vi "Voltage Ramp Text Out.vi"(1 "VoltageRamp":T2={"VISA Resource Name"="", "extra wait"=1, "start"=1e-12, "end"=0.002, "Sweep Time (H:M:S)"=1800.0, "Log Linear"=FALSE, "interval(sec)"=0.5, "Select instrument"=enum."Yokogawa GS200 Coarse"} {"interval(sec)" min=0.5 step=0.1; "Sweep Time (H:M:S)" format="%<%H:%M:%S>t"; "extra wait" min=0; "start" format="%#.7e"; "end" format="%#.7e"}) -> (0 "Command text":string[][](array[string]))   [LabVIEW 2021]
uses:
  VoltageRamp.ctl
  VoltageRamp Instrument.ctl
panel:
  out "Select instrument 2":T1
  out "Sweep Time (H:M:S)":dbl
  out "String Cluster":T3
  # "Voltage Ramp"
  # "Select\nInstrument"
  # "Instrument \nAddress"
  # "Log"
  # "End Voltage (V)"
  # "Sweep Time (HH:MM:SS)"
  # "Start Voltage (V)"
  # "Linear"
  # "seconds"
  # "Minimum Time Interval Between Two Points"
  # "seconds"
  # "AND wait extra"
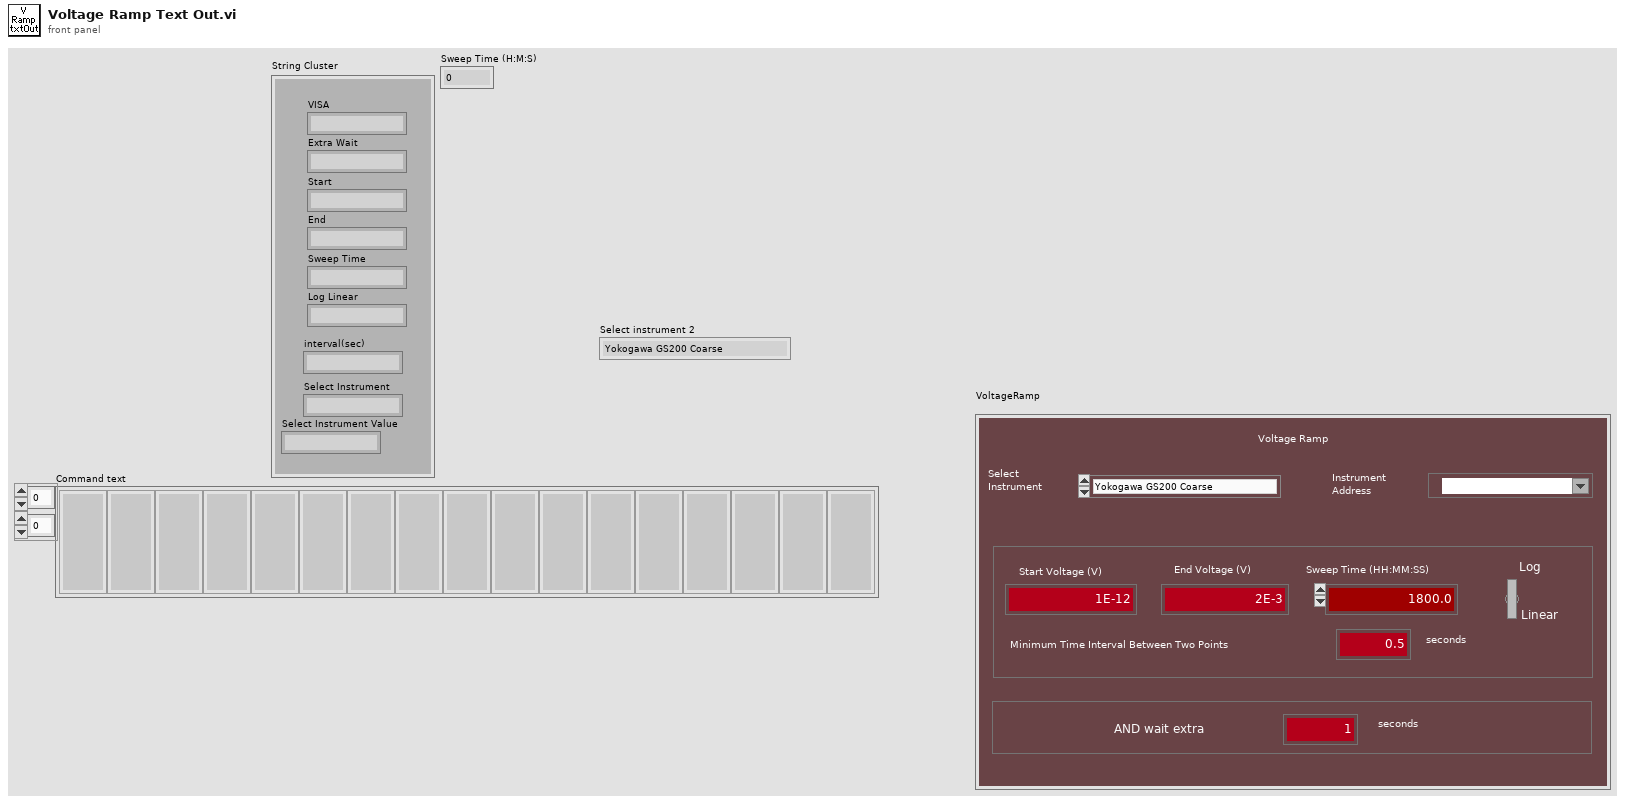
[diagram p1: front panel]
types:
  T1 = typedef "VoltageRamp Instrument.ctl" = enum16{"Yokogawa GS200 Coarse", "Keithley 24xx Coarse", "Keithley 230"}
  T2 = typedef "VoltageRamp.ctl" = cluster{"VISA Resource Name":refnum<visa-resource-name>, "extra wait":i32, "start":dbl, "end":dbl, "Sweep Time (H:M:S)":dbl, "Log Linear":bool, "interval(sec)":dbl, "Select instrument":T1}
  T3 = cluster{"VISA":string, "Extra Wait":string, "Start":string, "End":string, "Sweep Time":string, "Log Linear":string, "interval(sec)":string, "Select Instrument":string, "Select Instrument Value":string}
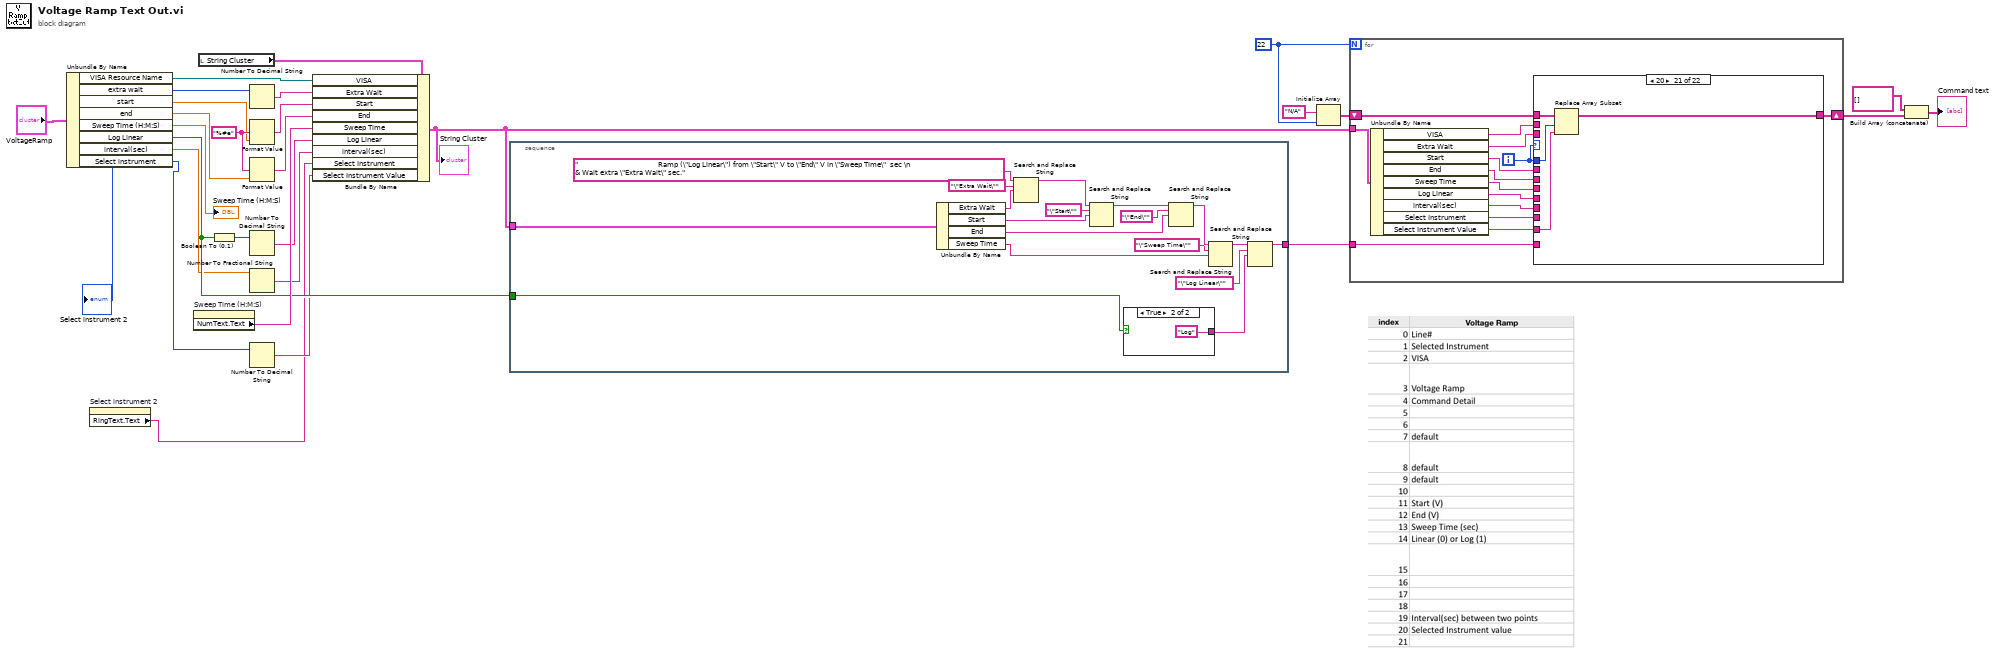
[diagram p0: block diagram]
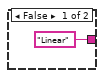
[diagram p2: hidden frame]
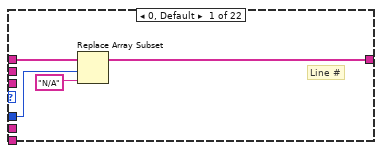
[diagram p3: hidden frame]
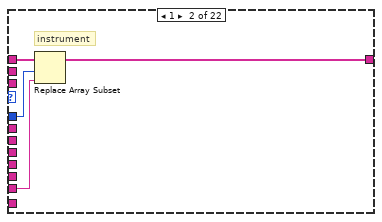
[diagram p4: hidden frame]
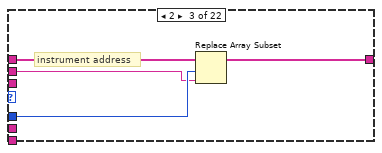
[diagram p5: hidden frame]
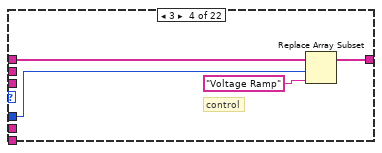
[diagram p6: hidden frame]
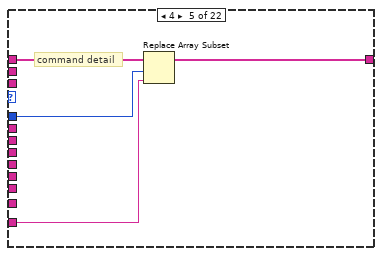
[diagram p7: hidden frame]
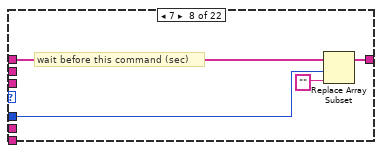
[diagram p10: hidden frame]
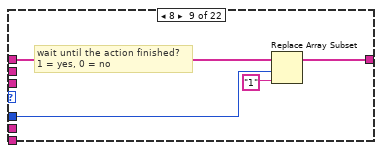
[diagram p11: hidden frame]
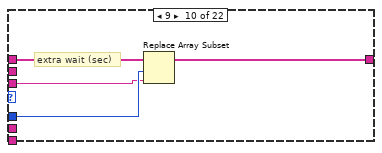
[diagram p12: hidden frame]
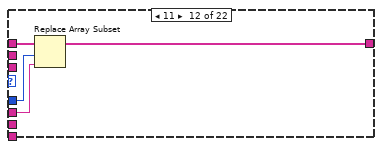
[diagram p14: hidden frame]
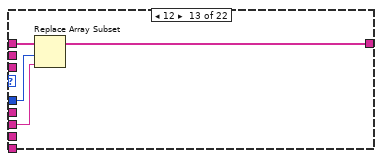
[diagram p15: hidden frame]
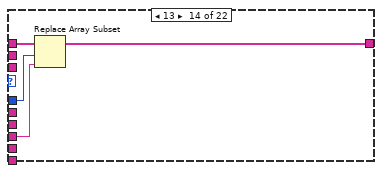
[diagram p16: hidden frame]
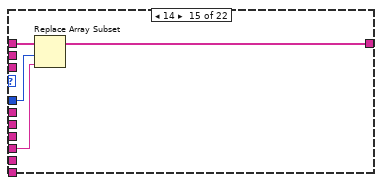
[diagram p17: hidden frame]
diagram:
  w17 = "%#e" ("format string")
  w25 = 22
  n1 = Unbundle By Name("VoltageRamp") -> ("VISA Resource Name"=w10:refnum<visa-resource-name>, "extra wait"=w12:i32, "start"=w15:dbl, "end"=w16:dbl, "Sweep Time (H:M:S)"=→"Sweep Time (H:M:S)":dbl, "Log Linear"=w8:bool, "interval(sec)"=w6:dbl, "Select instrument"=w1:T1)
  "Select instrument 2" <- w1
  n2 = property on="Select instrument 2" class="Enum (strict)"() -> ("RingText.Text"=w2:string)  [unwired: 2 in, 2 out]
  n3 = property on="Sweep Time (H:M:S)" class="DigNum (strict)"() -> ("NumText.Text"=w18:string)  [unwired: 2 in, 2 out]
  n4 = local read "String Cluster"() -> (w22:T3)
  n5 = Boolean To (0,1)(Boolean=w8) -> (0, 1=w9:i16)
  n6 = Number To Decimal String(number=w12) -> (decimal integer string=w11:string)  [unwired: 1 in]
  n7 = Format Value(format string=w17, value (0)=w15) -> (output string=w14:string)  [unwired: 1 in]
  n8 = Format Value(format string=w17, value (0)=w16) -> (output string=w13:string)  [unwired: 1 in]
  n9 = Number To Decimal String(number=w9) -> (decimal integer string=w7:string)  [unwired: 1 in]
  n10 = Number To Fractional String(number=w6) -> (F-format string=w5:string)  [unwired: 3 in]
  n11 = Number To Decimal String(number=w1) -> (decimal integer string=w4:string)  [unwired: 1 in]
  n12 = Bundle By Name(cluster=w22, "VISA"=w10, "Extra Wait"=w11, "Start"=w14, "End"=w13, "Sweep Time"=w18, "Log Linear"=w7, "interval(sec)"=w5, "Select Instrument"=w2, "Select Instrument Value"=w4) -> (w20:T3)
  "String Cluster" <- w20
  n13 = stacked-sequence {
    tunnel: [w32] -> w21
    tunnel: w20 -> [w38]
    tunnel: w8 -> [w29]
    frame #0 {
      n14 = Unbundle By Name(w38) -> ("Extra Wait"=w37:string, "Start"=w36:string, "End"=w35:string, "Sweep Time"=w34:string)
      n15 = Search and Replace String(input string="                                        Ramp (\"Log Linear\") from \"Start\" V to \"End\" V in \"Sweep Time\"  sec \n                                        & Wait extra \"Extra Wait\" sec.", search string="\"Extra Wait\"", replace string=w37) -> (result string=w44:string)  [unwired: 5 in, 3 out]
      n16 = Search and Replace String(input string=w44, search string="\"Start\"", replace string=w36) -> (result string=w45:string)  [unwired: 5 in, 3 out]
      n17 = case shown="True" w29 {
        tunnel: ["Linear" "Log"] -> w33
        frame False {
        }
        frame True {
        }
      }
      n18 = Search and Replace String(input string=w45, search string="\"End\"", replace string=w35) -> (result string=w46:string)  [unwired: 5 in, 3 out]
      n19 = Search and Replace String(input string=w46, search string="\"Sweep Time\"", replace string=w34) -> (result string=w31:string)  [unwired: 5 in, 3 out]
      n20 = Search and Replace String(input string=w31, search string="\"Log Linear\"", replace string=w33) -> (result string=w32:string)  [unwired: 5 in, 3 out]
    }
  }
  n21 = Initialize Array("N/A", w25) -> (w24:string[])
  n22 = for {
    N: w25 -> [_]
    shift-right: [w60] -> w23
    shift-left: w24 -> [w61]
    tunnel: w21 -> [w59]
    tunnel: w20 -> [w58]
    i -> [w62]
    n23 = Unbundle By Name(w58) -> ("VISA"=w55:string, "Extra Wait"=w54:string, "Start"=w57:string, "End"=w56:string, "Sweep Time"=w53:string, "Log Linear"=w50:string, "interval(sec)"=w51:string, "Select Instrument"=w52:string, "Select Instrument Value"=w49:string)
    n24 = case shown="20" w62 {
      tunnel: w62 -> [w65 w70 w74 w76 w81 _ _ w86 w90 w94 _ w99 w103 w109 w111 _ _ _ _ w118 w123 _]
      tunnel: w61 -> [w66 w69 w73 w77 w82 w83 w84 w88 w92 w96 w97 w100 w105 w107 w113 w114 w115 w116 w117 w121 w125 w126]
      tunnel: [w63 w68 w72 w75 w80 w83 w84 w87 w91 w95 w97 w101 w104 w106 w112 w114 w115 w116 w117 w120 w124 w126] -> w60
      tunnel: w59 -> [_ _ _ _ w79 _ _ _ _ _ _ _ _ _ _ _ _ _ _ _ _ _]
      tunnel: w57 -> [_ _ _ _ _ _ _ _ _ _ _ w98 _ _ _ _ _ _ _ _ _ _]
      tunnel: w56 -> [_ _ _ _ _ _ _ _ _ _ _ _ w102 _ _ _ _ _ _ _ _ _]
      tunnel: w55 -> [_ _ w71 _ _ _ _ _ _ _ _ _ _ _ _ _ _ _ _ _ _ _]
      tunnel: w54 -> [_ _ _ _ _ _ _ _ _ w93 _ _ _ _ _ _ _ _ _ _ _ _]
      tunnel: w53 -> [_ _ _ _ _ _ _ _ _ _ _ _ _ w108 _ _ _ _ _ _ _ _]
      tunnel: w51 -> [_ _ _ _ _ _ _ _ _ _ _ _ _ _ _ _ _ _ _ w119 _ _]
      tunnel: w52 -> [_ w67 _ _ _ _ _ _ _ _ _ _ _ _ _ _ _ _ _ _ _ _]
      tunnel: w50 -> [_ _ _ _ _ _ _ _ _ _ _ _ _ _ w110 _ _ _ _ _ _ _]
      tunnel: w49 -> [_ _ _ _ _ _ _ _ _ _ _ _ _ _ _ _ _ _ _ _ w122 _]
      frame 0, Default {
        # "Line #"
        n25 = Replace Array Subset(array=w66, new element="N/A", index=w65) -> (w63:string[])
      }
      frame 1 {
        # "instrument"
        n26 = Replace Array Subset(array=w69, new element=w67, index=w70) -> (w68:string[])
      }
      frame 2 {
        # "instrument address"
        n27 = Replace Array Subset(array=w73, new element=w71, index=w74) -> (w72:string[])
      }
      frame 3 {
        # "control"
        n28 = Replace Array Subset(array=w77, new element="Voltage Ramp", index=w76) -> (w75:string[])
      }
      frame 4 {
        # "command detail"
        n29 = Replace Array Subset(array=w82, new element=w79, index=w81) -> (w80:string[])
      }
      frame 5 {
        # "in  case 1"
      }
      frame 6 {
        # "in case 2"
      }
      frame 7 {
        # "wait before this command (sec)"
        n30 = Replace Array Subset(array=w88, new element="" ("new element/subarray"), index=w86) -> (w87:string[])
      }
      frame 8 {
        # "wait until the action finished?\n1 = yes, 0 = no"
        n31 = Replace Array Subset(array=w92, new element="1" ("new element/subarray"), index=w90) -> (w91:string[])
      }
      frame 9 {
        # "extra wait (sec)"
        n32 = Replace Array Subset(array=w96, new element=w93, index=w94) -> (w95:string[])
      }
      frame 10 {
      }
      frame 11 {
        n33 = Replace Array Subset(array=w100, new element=w98, index=w99) -> (w101:string[])
      }
      frame 12 {
        n34 = Replace Array Subset(array=w105, new element=w102, index=w103) -> (w104:string[])
      }
      frame 13 {
        n35 = Replace Array Subset(array=w107, new element=w108, index=w109) -> (w106:string[])
      }
      frame 14 {
        n36 = Replace Array Subset(array=w113, new element=w110, index=w111) -> (w112:string[])
      }
      frame 15 {
      }
      frame 16 {
      }
      frame 17 {
      }
      frame 18 {
      }
      frame 19 {
        n37 = Replace Array Subset(array=w121, new element=w119, index=w118) -> (w120:string[])
      }
      frame 20 {
        n38 = Replace Array Subset(array=w125, new element=w122, index=w123) -> (w124:string[])
      }
      frame 21 {
      }
    }
  }
  n39 = Build Array (concatenate)(string[][] [], w23) -> (→"Command text":string[][])
